vi "Maquina_2.vi"() -> ()   [LabVIEW 2016]
uses:
  Control2_Enum.ctl
panel:
  in  "F":bool
  in  "Paro":bool
  out "MD":bool
  out "MI":bool
  in  "S":bool
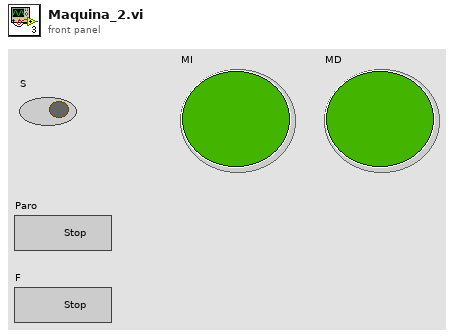
[diagram p1: front panel]
types:
  T1 = typedef "Control2_Enum.ctl" = enum16{"Avance", "Giro Izquierda", "Giro Derecha", "Espera"}
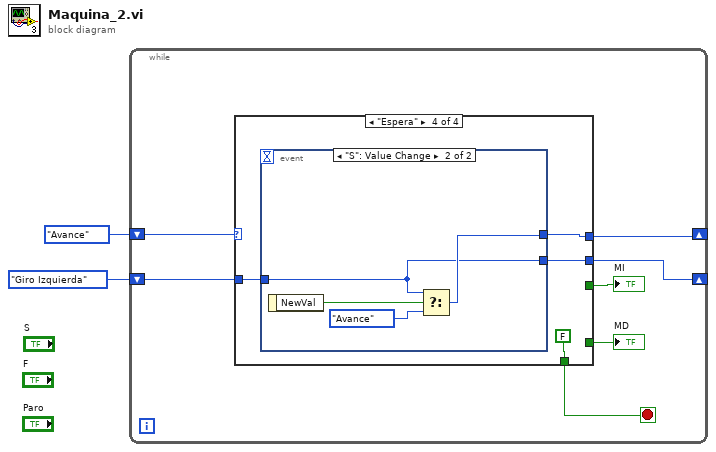
[diagram p0: block diagram]
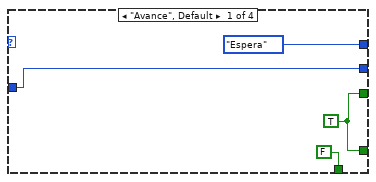
[diagram p2: hidden frame]
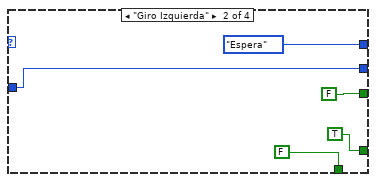
[diagram p3: hidden frame]
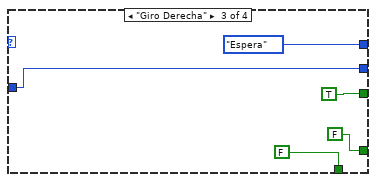
[diagram p4: hidden frame]
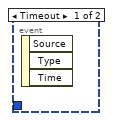
[diagram p5: hidden frame]
diagram:
  n1 = while {
    shift-right: [w5] -> _
    shift-left: Control2_Enum."Avance" -> [w9]
    shift-right: [w3] -> _
    shift-left: Control2_Enum."Giro Izquierda" -> [w4]
    stop <- w6 stop-if-true
    n2 = case shown="\"Espera\"" w9 {
      tunnel: [w13 FALSE TRUE _] -> w8
      tunnel: [w13 TRUE FALSE _] -> w7
      tunnel: [FALSE FALSE FALSE FALSE] -> w6
      tunnel: [Control2_Enum."Espera" Control2_Enum."Espera" Control2_Enum."Espera" w27] -> w5
      tunnel: w4 -> [w10 w14 w19 w26]
      tunnel: [w10 w14 w19 w25] -> w3
      frame "Avance", Default {
        w13 = TRUE
      }
      frame "Giro Izquierda" {
      }
      frame "Giro Derecha" {
      }
      frame "Espera" {
        n3 = event shown="[1] \"S\": Value Change" {
          selector: _ -> [_ _]
          dyn-events: _ -> [_ _]
          timeout: _ -> [_ _]
          tunnel: [_ w29] -> w27
          tunnel: w26 -> [_ w28]
          tunnel: [_ w28] -> w25
          event Timeout {
            n4 = event-data() -> ()  [unwired: 1 in, 3 out]
          }
          event "S": Value Change {
            n5 = event-data() -> ("NewVal"=w31:bool)  [unwired: 1 in]
            n6 = Select(t=w28, s=w31, f=Control2_Enum."Avance") -> (s? t:f=w29:T1)
          }
        }
      }
    }
    "MI" <- w8
    "MD" <- w7
  }
